vi "p1.vi"() -> ()   [LabVIEW 2021, in "d20.lvlib"]
uses:
  d20.lvlib
  Circular Buffer/Circular Buffer.lvclass
  AOC/AOC.lvlib
panel:
  out "index":i32
  in  "Example":string="1\n2\n-3\n3\n-2\n0\n4"
  in  "Example":bool=TRUE
  out "Answer":i64
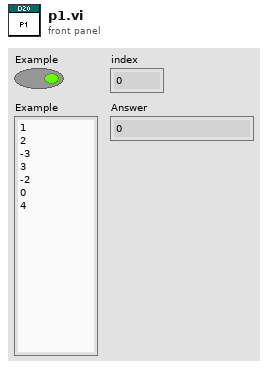
[diagram p1: front panel]
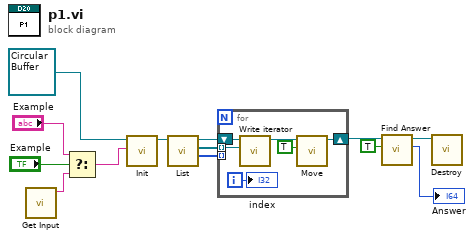
[diagram p0: block diagram]
diagram:
  n1 = call "Get Input.vi"() -> ("Input"=w13:string)  [unwired: 11 in]
  n2 = Select(t="Example", s="Example", f=w13) -> (s? t:f=w8:string)
  n3 = call "Init.vi"("Input"=w8, "Circular Buffer in"=refnum<class "Circular Buffer.lvclass"> refnum ("d20.lvlib:Circular Buffer.lvclass")) -> ("Circular Buffer out"=w1:refnum<class "Circular Buffer.lvclass">)  [unwired: 9 in]
  n4 = call "List.vi"("Circular Buffer in"=w1) -> ("Shift List"=w2:i64[], "Node List"=w7:refnum<data-value>[], "Circular Buffer out"=w9:refnum<class "Circular Buffer.lvclass">)  [unwired: 7 in, 1 out]
  n5 = for {
    tunnel: w7 -> [w17] mode=indexing
    shift-right: [w15] -> w6
    shift-left: w9 -> [w18]
    tunnel: w2 -> [_] mode=indexing
    i -> [w16]
    n6 = call "Write iterator.vi"("iterator"=w17, "Circular Buffer in"=w18) -> ("Circular Buffer out"=w19:refnum<class "Circular Buffer.lvclass">)  [unwired: 9 in]
    n7 = call "Move.vi"("P1"=TRUE, "Circular Buffer in"=w19) -> ("Circular Buffer out"=w15:refnum<class "Circular Buffer.lvclass">)  [unwired: 9 in]
    "index" <- w16
  }
  n8 = call "Find Answer.vi"("P1"=TRUE, "Circular Buffer in"=w6) -> ("Answer"=→"Answer":i64, "Circular Buffer out"=w5:refnum<class "Circular Buffer.lvclass">)  [unwired: 8 in]
  n9 = call "Destroy.vi"("Circular Buffer in"=w5) -> ()  [unwired: 11 in]
